vi "FORMAT.vi"(7 "mode":u8, 9 "Info":T1={"Sample Size"=1, "Data Type"=0, "Figures"=3, "Decimals"=0} {"Data Type" items=["DATA8", "DATA16", "DATA32", "DATAF"]}, 11 "Python in":string="import machine, utime\n\ntx = machine.Pin('Y9', machine.Pin.OUT)\nrx = machine.Pin('Y10', machine.Pin.IN)\ntx.value(b'\\x00')\nutime.sleep_ms(500)\ntx.value(1)\n\nuart = machine.UART(3)\nuart.init(baudrate=2400, bits=8, parity=None, stop=1)\n\nuart.write(0)\nuart.write(b'\\x40\\x23\\x9C')\nuart.write(b'\\x98\\x00\\x4C\\x69\\x67\\x68\\x74\\x00\\x00\\x00\\x39')\n") -> (3 "Python out":string="import machine, utime\n\ntx = machine.Pin('Y9', machine.Pin.OUT)\nrx = machine.Pin('Y10', machine.Pin.IN)\ntx.value(b'\\x00')\nutime.sleep_ms(500)\ntx.value(1)\n\nuart = machine.UART(3)\nuart.init(baudrate=2400, bits=8, parity=None, stop=1)\n\nuart.write(0)\nuart.write(b'\\x40\\x23\\x9C')\nuart.write(b'\\x98\\x00\\x4C\\x69\\x67\\x68\\x74\\x00\\x00\\x00\\x39')\nuart.write(b'\\x90\\x80\\x01\\x00\\x03\\x00\\xED')\n")   [LabVIEW 2016]
panel:
  out "bytes added":u8[](array[numeric])=[144, 128, 1, 0, 3, 0, 237] format="%.0x"
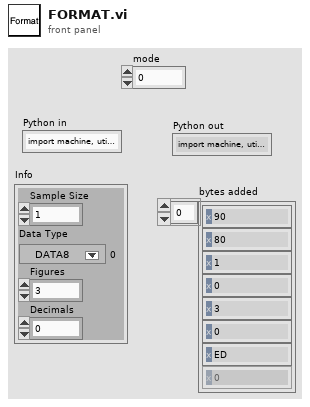
[diagram p1: front panel]
types:
  T1 = cluster{"Sample Size":u8, "Data Type":u8, "Figures":u8, "Decimals":u8}
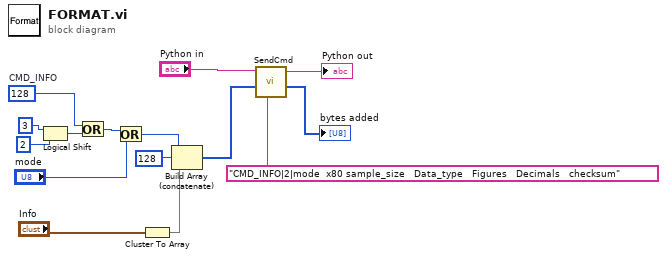
[diagram p0: block diagram]
diagram:
  w11 = u8 128  # CMD_INFO
  n1 = Logical Shift(y=i16 3, x=u8 2) -> (x << y=w10:u8)
  n2 = Or(x=w11, y=w10) -> (x .or. y?=w12:u8)
  n3 = Or(x=w12, y="mode") -> (x .or. y?=w3:u8)
  n4 = Cluster To Array(cluster="Info") -> (array=w5:u8[])
  n5 = Build Array (concatenate)(w3, u8 128 ("CMD_INFO"), w5) -> (w4:u8[])
  n6 = call "SendCmd.vi"("Comment"="CMD_INFO|2|mode  x80 sample_size   Data_type   Figures   Decimals   checksum", "Array In"=w4, "Python in"="Python in") -> ("Array Sent"=→"bytes added":u8[], "Python out"=→"Python out":string)  [unwired: 7 in]
